vi "Tab Engine.vi"(7 "Action":T5, 8 "error in (no error)":errorcluster, 11 "Variant in":variant) -> (0 "error out":errorcluster, 3 "Variant out":variant)   [LabVIEW 2018, in "Tab.lvlib"]
uses:
  Tab.lvlib
  Tab Action.ctl
  Tab Refnums.ctl
  Tab Mouse.ctl
  <vilib>/Utility/miscctls.llb/LVPoint32TypeDef.ctl
  Tab Add.ctl
  Tabs.ctl
panel:
  in  "StateData":T4
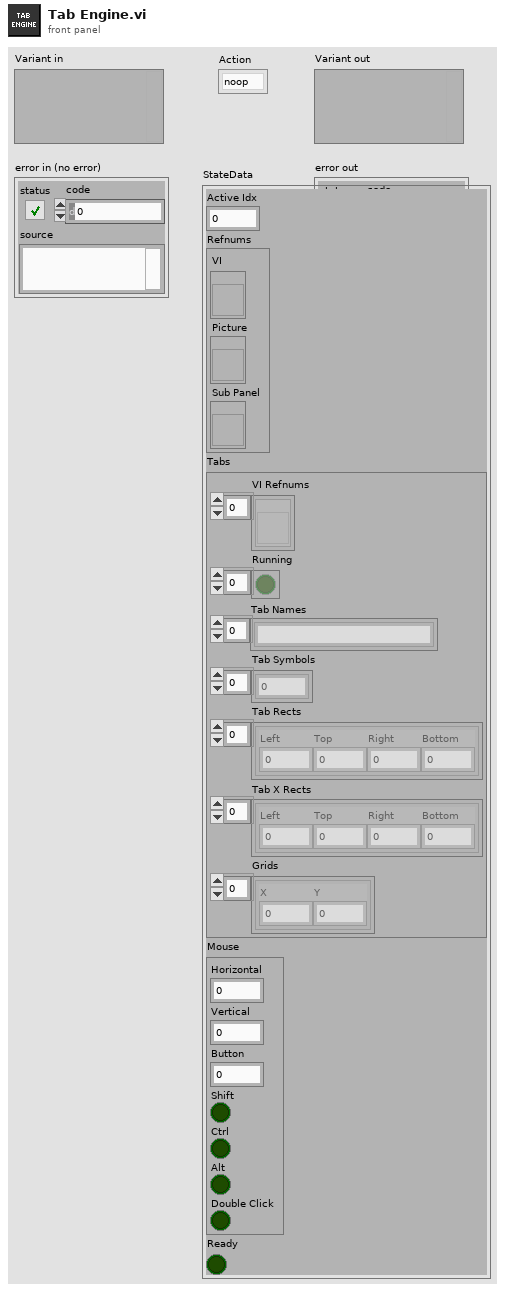
[diagram p1: front panel]
types:
  T1 = typedef "Tab.lvlib/Tab Refnums.ctl" = cluster{"VI":refnum<vi>, "Picture":refnum<vi>, "Sub Panel":refnum<vi>}
  T2 = typedef "Tab.lvlib/Tabs.ctl" = cluster{"VI Refnums":refnum<vi>[], "Running":bool[], "Tab Names":string[], "Tab Symbols":i32[], "Tab Rects":cluster{"Left":i16, "Top":i16, "Right":i16, "Bottom":i16}[], "Tab X Rects":cluster{"Left":i16, "Top":i16, "Right":i16, "Bottom":i16}[], "Grids":cluster{"X":i16, "Y":i16}[]}
  T3 = typedef "Tab.lvlib/Tab Mouse.ctl" = cluster{"Horizontal":i32, "Vertical":i32, "Button":u16, "Shift":bool, "Ctrl":bool, "Alt":bool, "Double Click":bool}
  T4 = cluster{"Active Idx":i32, "Refnums":T1, "Tabs":T2, "Mouse":T3, "Ready":bool}
  T5 = typedef "Tab.lvlib/Tab Action.ctl" = enum8{"noop", "new", "init", "close", "start", "render", "tab_add", "tab_change", "tab_hover", "tab_event", "tab_insert", "tab_popout", "tab_close", "theme_change", "resize"}
  T6 = typedef "LVPoint32TypeDef.ctl" = cluster{"Horizontal":i32, "Vertical":i32}
  T7 = typedef "Tab.lvlib/Tab Add.ctl" = cluster{"VI Path":path, "Name":string}
  T8 = cluster{"Left":i16, "Top":i16, "Right":i16, "Bottom":i16}
  T9 = cluster{"left":i16, "top":i16, "right":i16, "bottom":i16}[]
  T10 = cluster{"Left":i16, "Top":i16, "Right":i16, "Bottom":i16}[]
  T11 = enum32{"Invalid", "Standard", "Closed", "Hidden", "Minimized", "Maximized"}
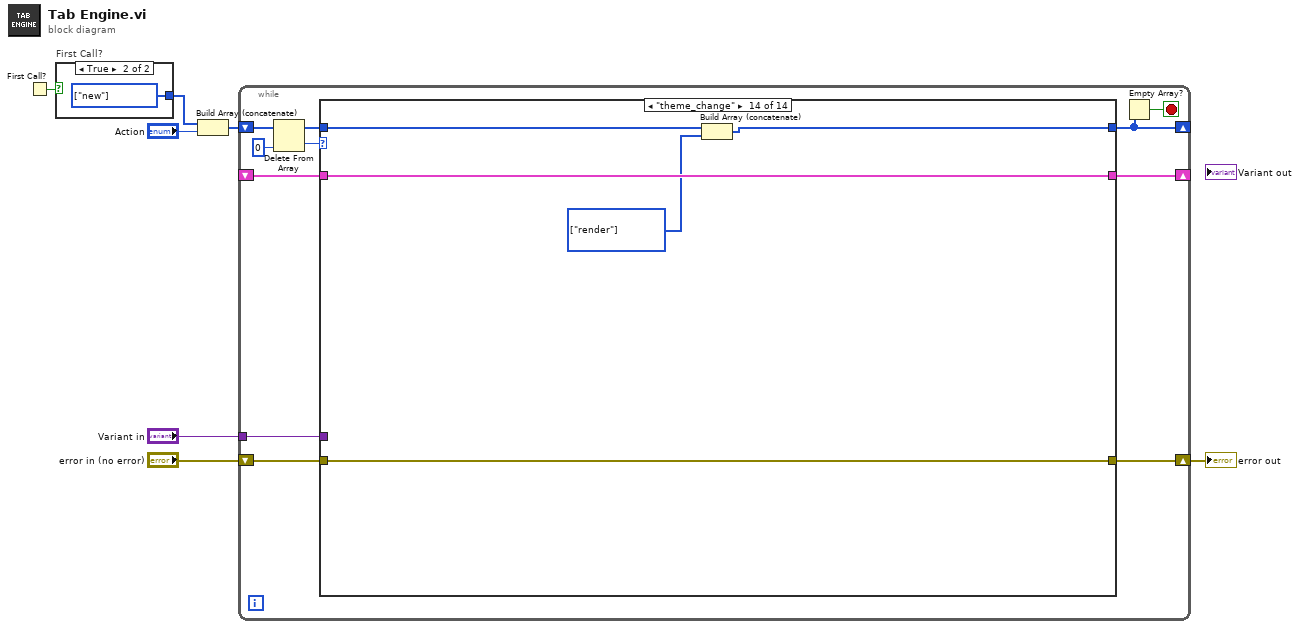
[diagram p0: block diagram]
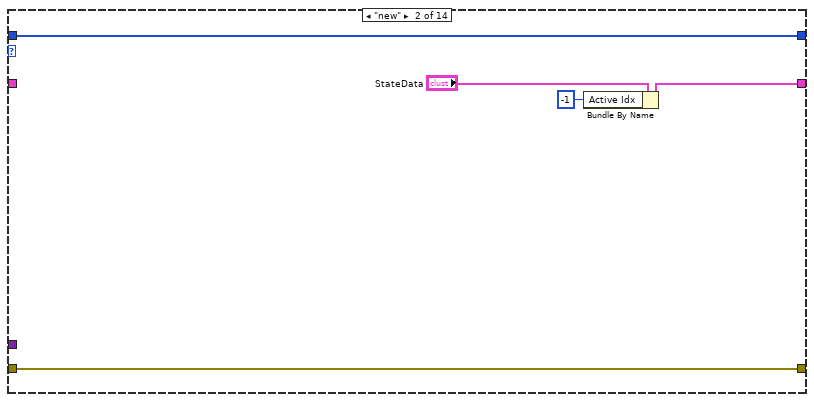
[diagram p4: hidden frame]
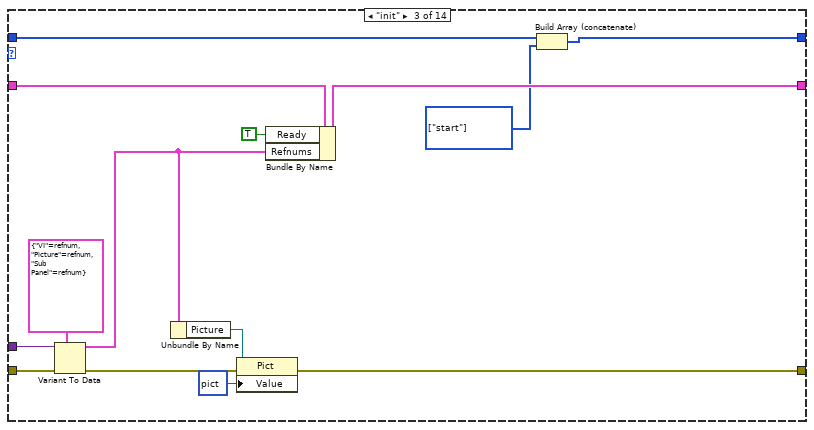
[diagram p5: hidden frame]
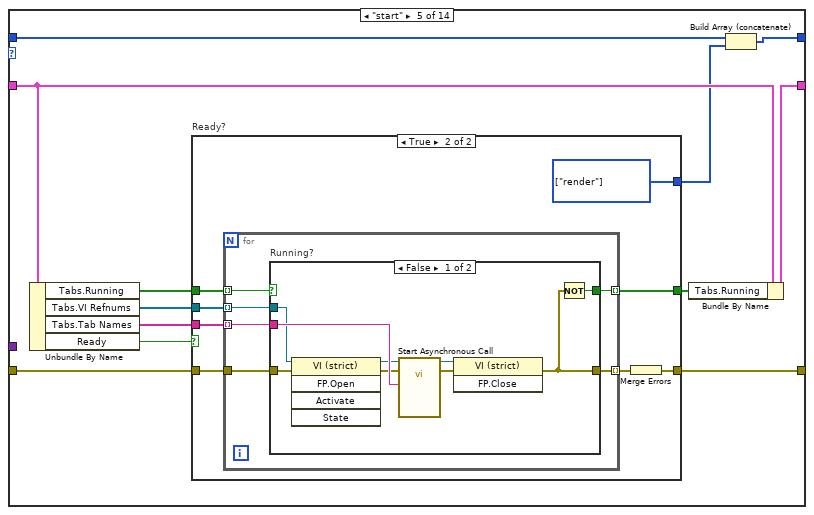
[diagram p7: hidden frame]
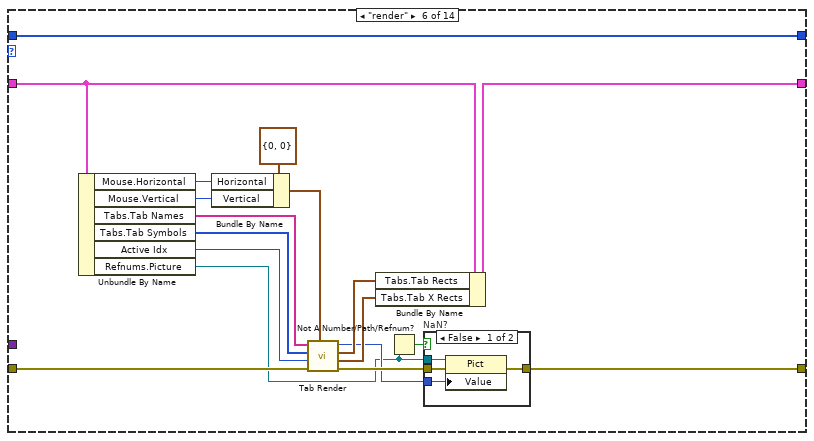
[diagram p10: hidden frame]
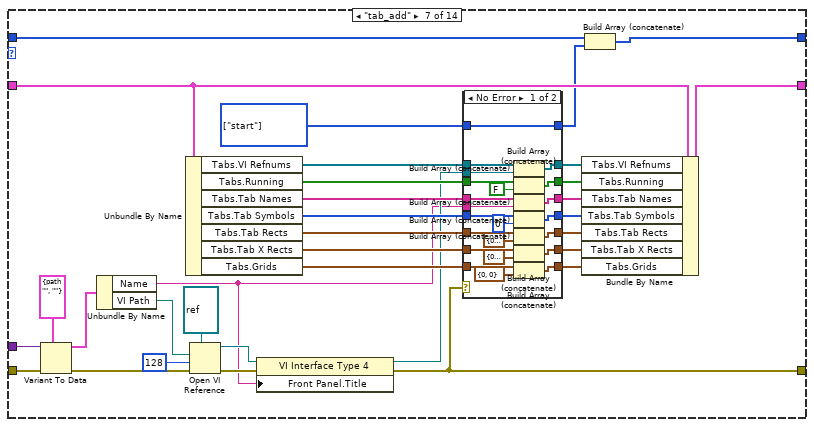
[diagram p12: hidden frame]
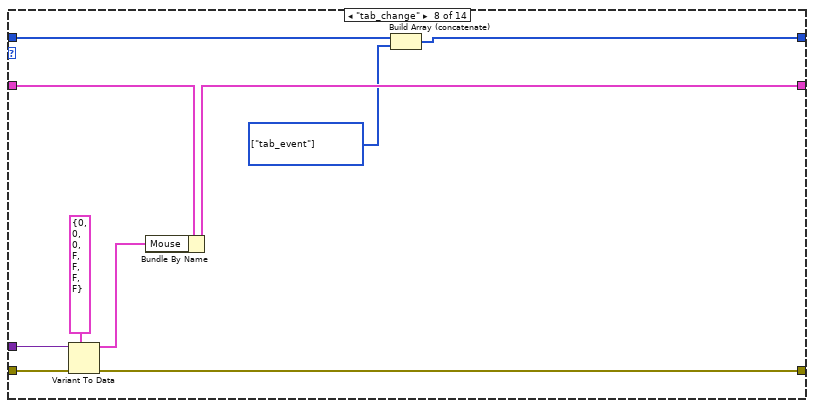
[diagram p14: hidden frame]
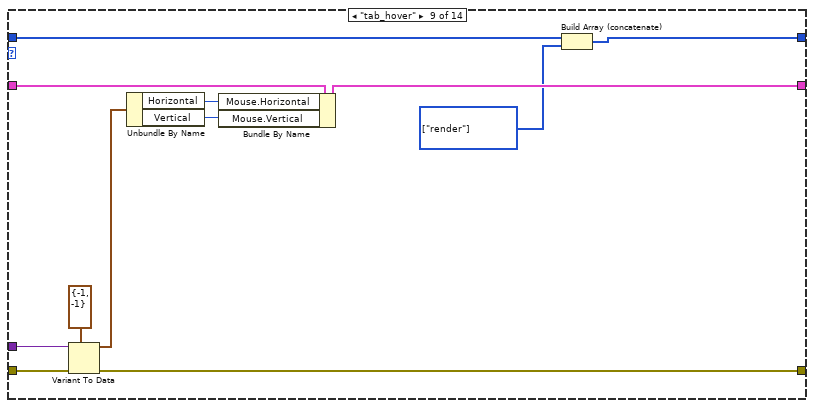
[diagram p15: hidden frame]
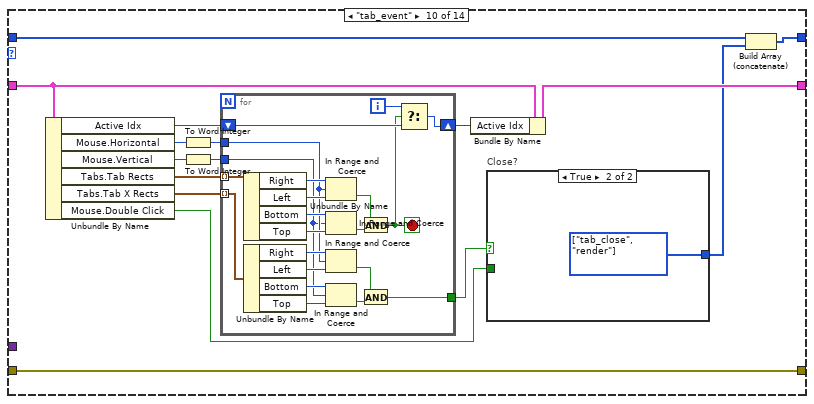
[diagram p16: hidden frame]
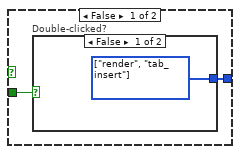
[diagram p17: hidden frame]
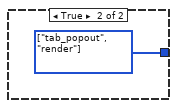
[diagram p18: hidden frame]
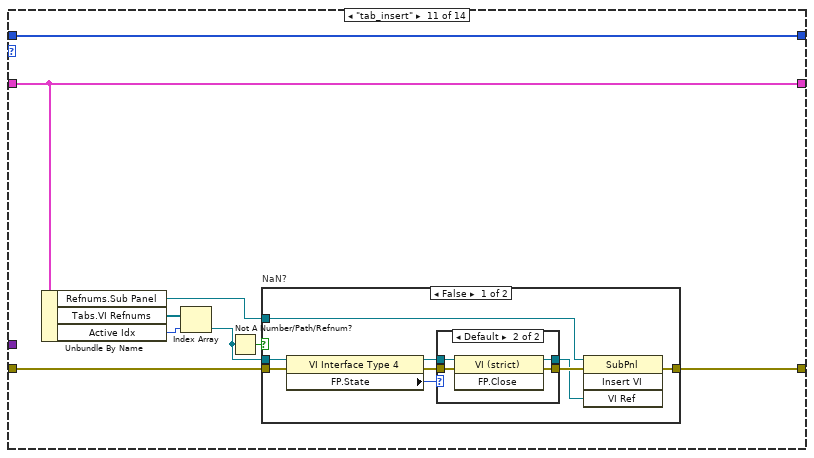
[diagram p19: hidden frame]
diagram:
  n1 = First Call?() -> (First Call?: T/F=w5:bool)
  n2 = case "First Call?" shown="True" w5 {
    tunnel: [_ w8] -> w6
    frame False {
    }
    frame True {
      w8 = T5[] [enum."new"] items=["noop", "new", "init", "close", "start", "render", "tab_add", "tab_change", "tab_hover", "tab_event", "tab_insert", "tab_popout", "tab_close", "theme_change", "resize"] ("appended array")
    }
  }
  n3 = Build Array (concatenate)(w6, "Action") -> (w4:T5[])
  n4 = while {
    shift-right: [w15] -> _
    shift-left: w4 -> [w19]
    shift-right: [w12] -> w2
    shift-left: "error in (no error)" -> [w13]
    shift-right: [w11] -> _
    shift-left: _ -> [w10]
    tunnel: "Variant in" -> [w9]
    stop <- w14 stop-if-true
    n5 = Delete From Array(array=w19, index=0) -> (deleted portion=w17:T5, array with subset deleted=w16:T5[])  [unwired: 1 in]
    n6 = case shown="\"theme_change\"" w17 {
      tunnel: [w21 w27 w30 w44 w46 w101 w127 w170 w180 w195 w241 w260 w269 w277] -> w15
      tunnel: w16 -> [w21 w27 w41 w44 w56 w101 w139 w178 w190 w206 w241 w260 w269 w280]
      tunnel: w13 -> [w22 w26 w40 w43 w55 w98 w138 w177 w189 w205 w236 w259 w264 w279]
      tunnel: [w22 w26 w33 w43 w52 w87 w110 w176 w187 w205 w234 w259 w262 w279] -> w12
      tunnel: [w20 w24 w35 w42 w53 w90 w128 w173 w185 w197 w240 w258 w268 w278] -> w11
      tunnel: w10 -> [w20 _ w39 w42 w54 w100 w129 w171 w188 w204 w240 w258 w268 w278]
      tunnel: w9 -> [_ _ w37 _ _ _ w137 w175 w186 _ _ _ _ _]
      frame "noop", Default {
      }
      frame "new" {
        n7 = Bundle By Name(cluster="StateData", "Active Idx"=-1) -> (w24:T4)
      }
      frame "init" {
        w29 = T5[] [enum."start"] items=["noop", "new", "init", "close", "start", "render", "tab_add", "tab_change", "tab_hover", "tab_event", "tab_insert", "tab_popout", "tab_close", "theme_change", "resize"] ("array")
        n8 = Variant To Data(error in=w40, type=T1 {"VI"=refnum, "Picture"=refnum, "Sub Panel"=refnum} ("Refnums"), Variant=w37) -> (data=w34:T1, error out=w38:errorcluster)
        n9 = Unbundle By Name(w34) -> ("Picture"=w32:refnum<vi>)
        n10 = property class="Pict"(reference=w32, error in=w38, "Value"=picture data[5B]) -> (error out=w33:errorcluster)  [unwired: 1 out]
        n11 = Bundle By Name(cluster=w39, "Ready"=TRUE, "Refnums"=w34) -> (w35:T4)
        n12 = Build Array (concatenate)(w41, w29) -> (w30:T5[])
      }
      frame "close" {
      }
      frame "start" {
        n13 = Unbundle By Name(w54) -> ("Tabs.Running"=w50:bool[], "Tabs.VI Refnums"=w51:refnum<vi>[], "Tabs.Tab Names"=w49:string[], "Ready"=w48:bool)
        n14 = case "Ready?" shown="True" w48 {
          tunnel: w55 -> [w58 w66]
          tunnel: [w58 w60] -> w52
          tunnel: w51 -> [_ w64]
          tunnel: w50 -> [w57 w63]
          tunnel: w49 -> [_ w62]
          tunnel: [w57 w61] -> w47
          tunnel: [_ w59] -> w45
          frame False {
          }
          frame True {
            w59 = T5[] [enum."render"] items=["noop", "new", "init", "close", "start", "render", "tab_add", "tab_change", "tab_hover", "tab_event", "tab_insert", "tab_popout", "tab_close", "theme_change", "resize"] ("array")
            n15 = for {
              tunnel: w64 -> [w71] mode=indexing
              tunnel: w66 -> [w72]
              tunnel: [w70] -> w65 mode=indexing
              tunnel: w63 -> [w68] mode=indexing
              tunnel: w62 -> [w69] mode=indexing
              tunnel: [w67] -> w61 mode=indexing
              n16 = case "Running?" shown="False" w68 {
                selector: w68 -> [_ w82]
                tunnel: w72 -> [w81 w83]
                tunnel: w71 -> [w76 _]
                tunnel: [w74 w83] -> w70
                tunnel: w69 -> [w79 _]
                tunnel: [w78 w82] -> w67
                frame False {
                  n17 = invoke class="VI (strict)" method="FP.Open"(reference=w76, error in=w81) -> (reference out=w75:refnum<vi>, error out=w77:errorcluster)  [unwired: 3 in, 3 out]
                  n18 = call-by-ref "Start Asynchronous Call"(reference=w75, error in=w77, "Name"=w79) -> (reference out=w73:refnum<vi>, error out=w80:errorcluster)  [unwired: 11 in]
                  n19 = invoke class="VI (strict)" method="FP.Close"(reference=w73, error in=w80) -> (error out=w74:errorcluster)  [unwired: 1 in, 2 out]
                  n20 = Not(x=w74) -> (.not. x?=w78:bool)
                }
                frame True {
                }
              }
            }
            n21 = Merge Errors(w65) -> (w60:errorcluster)
          }
        }
        n22 = Bundle By Name(cluster=w54, "Tabs.Running"=w47) -> (w53:T4)
        n23 = Build Array (concatenate)(w56, w45) -> (w46:T5[])
      }
      frame "render" {
        n24 = Unbundle By Name(w100) -> ("Mouse.Horizontal"=w94:i32, "Mouse.Vertical"=w93:i32, "Tabs.Tab Names"=w97:string[], "Tabs.Tab Symbols"=w92:i32[], "Active Idx"=w91:i32, "Refnums.Picture"=w85:refnum<vi>)
        n25 = Bundle By Name(cluster=T6 {"Horizontal"=0, "Vertical"=0} ("Mouse Coords"), "Horizontal"=w94, "Vertical"=w93) -> (w95:T6)
        n26 = call "Tab Render.vi"("Mouse Coords"=w95, "error in (no error)"=w98, "Active Idx (-1)"=w91, "Tab Symbols"=w92, "Tab Names"=w97) -> ("error out"=w99:errorcluster, "Tab X Rects"=w88:T9, "Tab Rects"=w89:T9, "Picture"=w86:picture)  [unwired: 3 in]
        n27 = Bundle By Name(cluster=w100, "Tabs.Tab Rects"=w89, "Tabs.Tab X Rects"=w88) -> (w90:T4)
        n28 = Not A Number/Path/Refnum?(number/path/refnum=w85) -> (NaN/Path/Refnum?=w84:bool)
        n29 = case "NaN?" shown="False" w84 {
          tunnel: w99 -> [w105 w106]
          tunnel: [w104 w106] -> w87
          tunnel: w86 -> [w103 _]
          tunnel: w85 -> [w102 _]
          frame False {
            n30 = property class="Pict"(reference=w102, error in=w105, "Value"=w103) -> (error out=w104:errorcluster)  [unwired: 1 out]
          }
          frame True {
          }
        }
      }
      frame "tab_add" {
        w126 = T5[] [enum."start"] items=["noop", "new", "init", "close", "start", "render", "tab_add", "tab_change", "tab_hover", "tab_event", "tab_insert", "tab_popout", "tab_close", "theme_change", "resize"] ("array")
        n31 = Variant To Data(error in=w138, type=T7 {"VI Path"=path "", "Name"=""} ("Tab Add"), Variant=w137) -> (data=w130:T7, error out=w131:errorcluster)
        n32 = Unbundle By Name(w130) -> ("Name"=w107:string, "VI Path"=w135:path)
        n33 = Unbundle By Name(w129) -> ("Tabs.VI Refnums"=w133:refnum<vi>[], "Tabs.Running"=w121:bool[], "Tabs.Tab Names"=w119:string[], "Tabs.Tab Symbols"=w117:i32[], "Tabs.Tab Rects"=w115:T10, "Tabs.Tab X Rects"=w113:T10, "Tabs.Grids"=w111:cluster{"X":i16, "Y":i16}[])
        n34 = Open VI Reference(type specifier VI Refnum (for type only)=refnum<vi> refnum, vi path=w135, options=128, error in (no error)=w131) -> (vi reference=w109:refnum<vi>, error out=w124:errorcluster)  [unwired: 2 in]
        n35 = property class="VI Interface Type 4"(reference=w109, error in=w124, "Front Panel.Title"=w107) -> (reference out=w108:refnum<vi>, error out=w110:errorcluster)
        n36 = case shown="No Error" w110 {
          tunnel: w133 -> [w158 w168]
          tunnel: [w161 w168] -> w132
          tunnel: w108 -> [w160 _]
          tunnel: [w159 _] -> w125
          tunnel: w126 -> [w159 _]
          tunnel: [w146 w167] -> w122
          tunnel: w121 -> [w157 w167]
          tunnel: [w147 w166] -> w120
          tunnel: w119 -> [w156 w166]
          tunnel: [w148 w165] -> w118
          tunnel: w117 -> [w155 w165]
          tunnel: [w149 w164] -> w116
          tunnel: w115 -> [w154 w164]
          tunnel: [w150 w163] -> w114
          tunnel: w113 -> [w153 w163]
          tunnel: [w151 w162] -> w112
          tunnel: w111 -> [w152 w162]
          tunnel: w107 -> [w140 _]
          frame No Error {
            n37 = Build Array (concatenate)(w158, w160) -> (w161:refnum<vi>[])
            n38 = Build Array (concatenate)(w157, FALSE ("Boolean")) -> (w146:bool[])
            n39 = Build Array (concatenate)(w156, w140) -> (w147:string[])
            n40 = Build Array (concatenate)(w155, 0 ("array")) -> (w148:i32[])
            n41 = Build Array (concatenate)(w154, T8 {"Left"=0, "Top"=0, "Right"=0, "Bottom"=0} ("array")) -> (w149:T10)
            n42 = Build Array (concatenate)(w153, T8 {"Left"=0, "Top"=0, "Right"=0, "Bottom"=0} ("array")) -> (w150:T10)
            n43 = Build Array (concatenate)(w152, cluster{"X":i16, "Y":i16} {"X"=0, "Y"=0} ("array")) -> (w151:cluster{"X":i16, "Y":i16}[])
          }
          frame Error {
          }
        }
        n44 = Bundle By Name(cluster=w129, "Tabs.VI Refnums"=w132, "Tabs.Running"=w122, "Tabs.Tab Names"=w120, "Tabs.Tab Symbols"=w118, "Tabs.Tab Rects"=w116, "Tabs.Tab X Rects"=w114, "Tabs.Grids"=w112) -> (w128:T4)
        n45 = Build Array (concatenate)(w139, w125) -> (w127:T5[])
      }
      frame "tab_change" {
        w169 = T5[] [enum."tab_event"] items=["noop", "new", "init", "close", "start", "render", "tab_add", "tab_change", "tab_hover", "tab_event", "tab_insert", "tab_popout", "tab_close", "theme_change", "resize"] ("array")
        n46 = Variant To Data(error in=w177, type=T3 {"Horizontal"=0, "Vertical"=0, "Button"=0, "Shift"=FALSE, "Ctrl"=FALSE, "Alt"=FALSE, "Double Click"=FALSE} ("Mouse"), Variant=w175) -> (data=w172:T3, error out=w176:errorcluster)
        n47 = Bundle By Name(cluster=w171, "Mouse"=w172) -> (w173:T4)
        n48 = Build Array (concatenate)(w178, w169) -> (w170:T5[])
      }
      frame "tab_hover" {
        w179 = T5[] [enum."render"] items=["noop", "new", "init", "close", "start", "render", "tab_add", "tab_change", "tab_hover", "tab_event", "tab_insert", "tab_popout", "tab_close", "theme_change", "resize"] ("array")
        n49 = Variant To Data(error in=w189, type=T6 {"Horizontal"=-1, "Vertical"=-1} ("Coords"), Variant=w186) -> (data=w184:T6, error out=w187:errorcluster)
        n50 = Unbundle By Name(w184) -> ("Horizontal"=w182:i32, "Vertical"=w181:i32)
        n51 = Bundle By Name(cluster=w188, "Mouse.Horizontal"=w182, "Mouse.Vertical"=w181) -> (w185:T4)
        n52 = Build Array (concatenate)(w190, w179) -> (w180:T5[])
      }
      frame "tab_event" {
        n53 = Unbundle By Name(w204) -> ("Active Idx"=w200:i32, "Mouse.Horizontal"=w203:i32, "Mouse.Vertical"=w202:i32, "Tabs.Tab Rects"=w201:T10, "Tabs.Tab X Rects"=w193:T10, "Mouse.Double Click"=w191:bool)
        n54 = To Word Integer(number=w203) -> (16bit integer=w198:i16)
        n55 = To Word Integer(number=w202) -> (16bit integer=w199:i16)
        n56 = for {
          tunnel: w198 -> [w216]
          tunnel: w199 -> [w215]
          tunnel: w201 -> [w232] mode=indexing
          shift-right: [w227] -> w196
          shift-left: w200 -> [w229]
          tunnel: w193 -> [w214] mode=indexing
          tunnel: [w212] -> w192
          i -> [w228]
          stop <- w213 stop-if-true
          n57 = Unbundle By Name(w232) -> ("Right"=w226:i16, "Left"=w225:i16, "Bottom"=w224:i16, "Top"=w223:i16)
          n58 = Unbundle By Name(w214) -> ("Right"=w219:i16, "Left"=w220:i16, "Bottom"=w221:i16, "Top"=w222:i16)
          n59 = In Range and Coerce(upper limit=w226, x=w216, lower limit=w225) -> (In Range?=w230:bool)  [unwired: 1 out]
          n60 = In Range and Coerce(upper limit=w224, x=w215, lower limit=w223) -> (In Range?=w231:bool)  [unwired: 1 out]
          n61 = In Range and Coerce(upper limit=w219, x=w216, lower limit=w220) -> (In Range?=w218:bool)  [unwired: 1 out]
          n62 = In Range and Coerce(upper limit=w221, x=w215, lower limit=w222) -> (In Range?=w217:bool)  [unwired: 1 out]
          n63 = And(x=w230, y=w231) -> (x .and. y?=w213:bool)
          n64 = And(x=w218, y=w217) -> (x .and. y?=w212:bool)
          n65 = Select(t=w228, s=w213, f=w229) -> (s? t:f=w227:i32)
        }
        n66 = Bundle By Name(cluster=w204, "Active Idx"=w196) -> (w197:T4)
        n67 = case "Close?" shown="True" w192 {
          tunnel: [w208 w211] -> w194
          tunnel: w191 -> [w207 _]
          frame False {
            n68 = case "Double-clicked?" shown="False" w207 {
              tunnel: [w209 w210] -> w208
              frame False {
                w209 = T5[] [enum."render", enum."tab_insert"] items=["noop", "new", "init", "close", "start", "render", "tab_add", "tab_change", "tab_hover", "tab_event", "tab_insert", "tab_popout", "tab_close", "theme_change", "resize"] ("array")
              }
              frame True {
                w210 = T5[] [enum."tab_popout", enum."render"] items=["noop", "new", "init", "close", "start", "render", "tab_add", "tab_change", "tab_hover", "tab_event", "tab_insert", "tab_popout", "tab_close", "theme_change", "resize"] ("array")
              }
            }
          }
          frame True {
            w211 = T5[] [enum."tab_close", enum."render"] items=["noop", "new", "init", "close", "start", "render", "tab_add", "tab_change", "tab_hover", "tab_event", "tab_insert", "tab_popout", "tab_close", "theme_change", "resize"] ("array")
          }
        }
        n69 = Build Array (concatenate)(w206, w194) -> (w195:T5[])
      }
      frame "tab_insert" {
        n70 = Unbundle By Name(w240) -> ("Refnums.Sub Panel"=w233:refnum<vi>, "Tabs.VI Refnums"=w239:refnum<vi>[], "Active Idx"=w238:i32)
        n71 = Index Array(array=w239, index=w238) -> (element=w235:refnum<vi>)
        n72 = Not A Number/Path/Refnum?(number/path/refnum=w235) -> (NaN/Path/Refnum?=w237:bool)
        n73 = case "NaN?" shown="False" w237 {
          tunnel: w236 -> [w250 w257]
          tunnel: w233 -> [w249 _]
          tunnel: [w242 w257] -> w234
          tunnel: w235 -> [w244 _]
          frame False {
            n74 = property class="VI Interface Type 4"(reference=w244, error in=w250) -> (reference out=w246:refnum<vi>, error out=w248:errorcluster, "FP.State"=w245:T11)
            n75 = case shown="Default" w245 {
              tunnel: w248 -> [w252 w256]
              tunnel: [w252 w255] -> w247
              tunnel: w246 -> [w251 w254]
              tunnel: [w251 w253] -> w243
              frame "Invalid", "Closed" {
              }
              frame Default {
                n76 = invoke class="VI (strict)" method="FP.Close"(reference=w254, error in=w256) -> (reference out=w253:refnum<vi>, error out=w255:errorcluster)  [unwired: 1 in, 1 out]
              }
            }
            n77 = invoke class="SubPnl" method="Insert VI"(reference=w249, error in=w247, "VI Ref"=w243) -> (error out=w242:errorcluster)  [unwired: 1 in, 3 out]
          }
          frame True {
          }
        }
      }
      frame "tab_close" {
      }
      frame "tab_popout" {
        n78 = Unbundle By Name(w268) -> ("Refnums.Sub Panel"=w261:refnum<vi>, "Tabs.VI Refnums"=w267:refnum<vi>[], "Active Idx"=w266:i32)
        n79 = Index Array(array=w267, index=w266) -> (element=w263:refnum<vi>)
        n80 = Not A Number/Path/Refnum?(number/path/refnum=w263) -> (NaN/Path/Refnum?=w265:bool)
        n81 = case "NaN?" shown="False" w265 {
          tunnel: w264 -> [w272 w275]
          tunnel: w261 -> [w271 _]
          tunnel: [w273 w275] -> w262
          tunnel: w263 -> [w270 _]
          frame False {
            n82 = invoke class="SubPnl" method="Remove VI"(reference=w271, error in=w272) -> (error out=w274:errorcluster)  [unwired: 1 in, 2 out]
            n83 = invoke class="VI (strict)" method="FP.Open"(reference=w270, error in=w274) -> (error out=w273:errorcluster)  [unwired: 3 in, 4 out]
          }
          frame True {
          }
        }
      }
      frame "theme_change" {
        w276 = T5[] [enum."render"] items=["noop", "new", "init", "close", "start", "render", "tab_add", "tab_change", "tab_hover", "tab_event", "tab_insert", "tab_popout", "tab_close", "theme_change", "resize"] ("array")
        n84 = Build Array (concatenate)(w280, w276) -> (w277:T5[])
      }
    }
    n85 = Empty Array?(array=w15) -> (empty?=w14:bool)
  }
  "error out" <- w2
